vi "Oscilloscope.vi"() -> ()   [LabVIEW 2020]
uses:
  <vilib>/Utility/file.llb/Read Delimited Spreadsheet (DBL).vi
  <vilib>/express/express analysis/Spectral/Block/exnSpectralBlock spectral measurements RMS poly.vi
  <vilib>/express/express analysis/Spectral/Block/exnSpectralBlock spectral measurements RMS array WFM.vi
  <vilib>/express/express analysis/Spectral/XNode/ExpressSpectralMeasurementsBlockNode.xnode
panel:
  in  "Auto":bool
  in  "Amplitude/div":i32(knob)=10 scale=1.0..6.0
  in  "WAV Select":path
  in  "CSV Select":path
  in  "Save Image":bool
  in  "Channel":bool
  in  "High Cut Off":dbl(knob)=20000.0 min=1.0 scale=1.0..20000.0
  out "Moving Average Enable":bool
  in  "Moving Average Enable":bool
  in  "Moving Average\nWindow Size":u16(ring) items=["4", "8", "16"]
  in  "Reset":bool
  in  "Input Select":bool
  in  "stop":bool
  in  "Filter Order":i16(knob)=1 scale=1.0..5.0
  in  "Pause/Continue":bool
  in  "Tab Control":enum32{"Time", "FFT"}(tab)
  out "Waveform Chart":dbl(graph)
  out "Waveform Graph":cluster{"f0":dbl, "df":dbl, "magnitude":dbl[]}[](graph)
  in  "Period (ms)":dbl(knob)=10.0 scale=1.0..100.0
  out "Frequency (Hz)":dbl
  in  "Amplitude Control":dbl(knob)=1.0 min=1.0 scale=1.0..1000.0
  in  "Offset":i32(knob) scale=-10.0..10.0
  in  "Orig or not":bool=TRUE
  out "Original":bool
  in  "Filter or not":bool
  in  "Filter Select":u16(ring) items=["Lowpass", "Highpass", "Bandpass", "Bandstop", "Smoothing"]
  in  "Low Cut Off":dbl(knob)=1.0 min=1.0 scale=1.0..20000.0
  out "Filter Enable":bool
  in  "Phase Control":dbl(knob) scale=-360.0..360.0
  out "Pk-Pk":dbl
  out "RMS":dbl
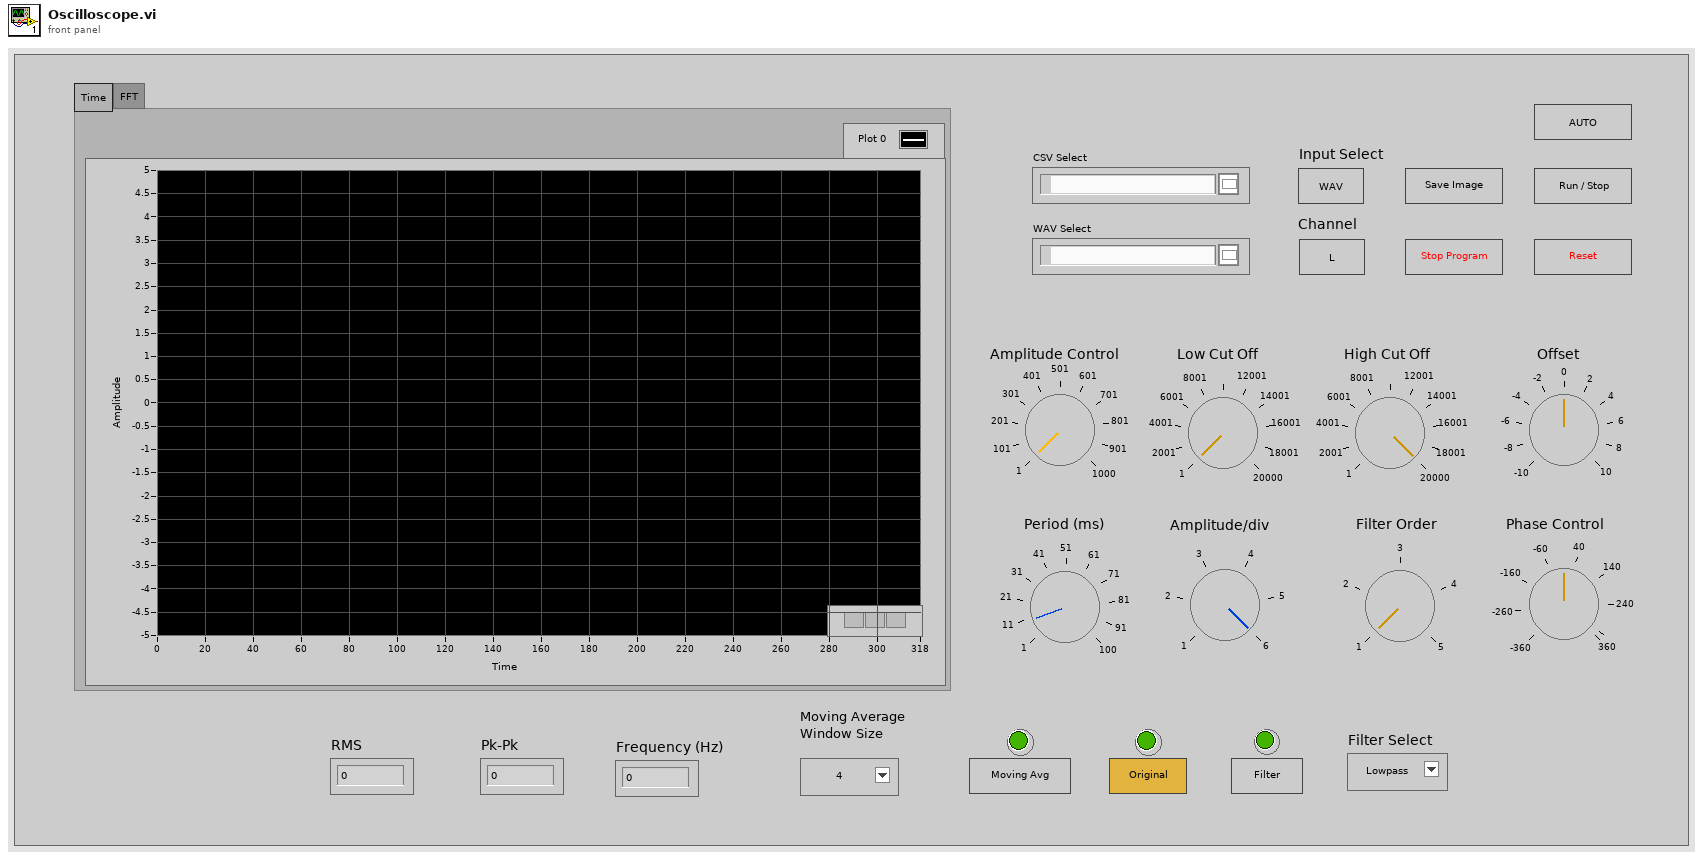
[diagram p1: front panel]
types:
  T1 = cluster{"averaging mode":u16, "weighting mode":u16, "number of averages":u32}
  T2 = cluster{"dB On (F)":bool, "unwrap phase (F)":bool, "convert to degree (F)":bool}
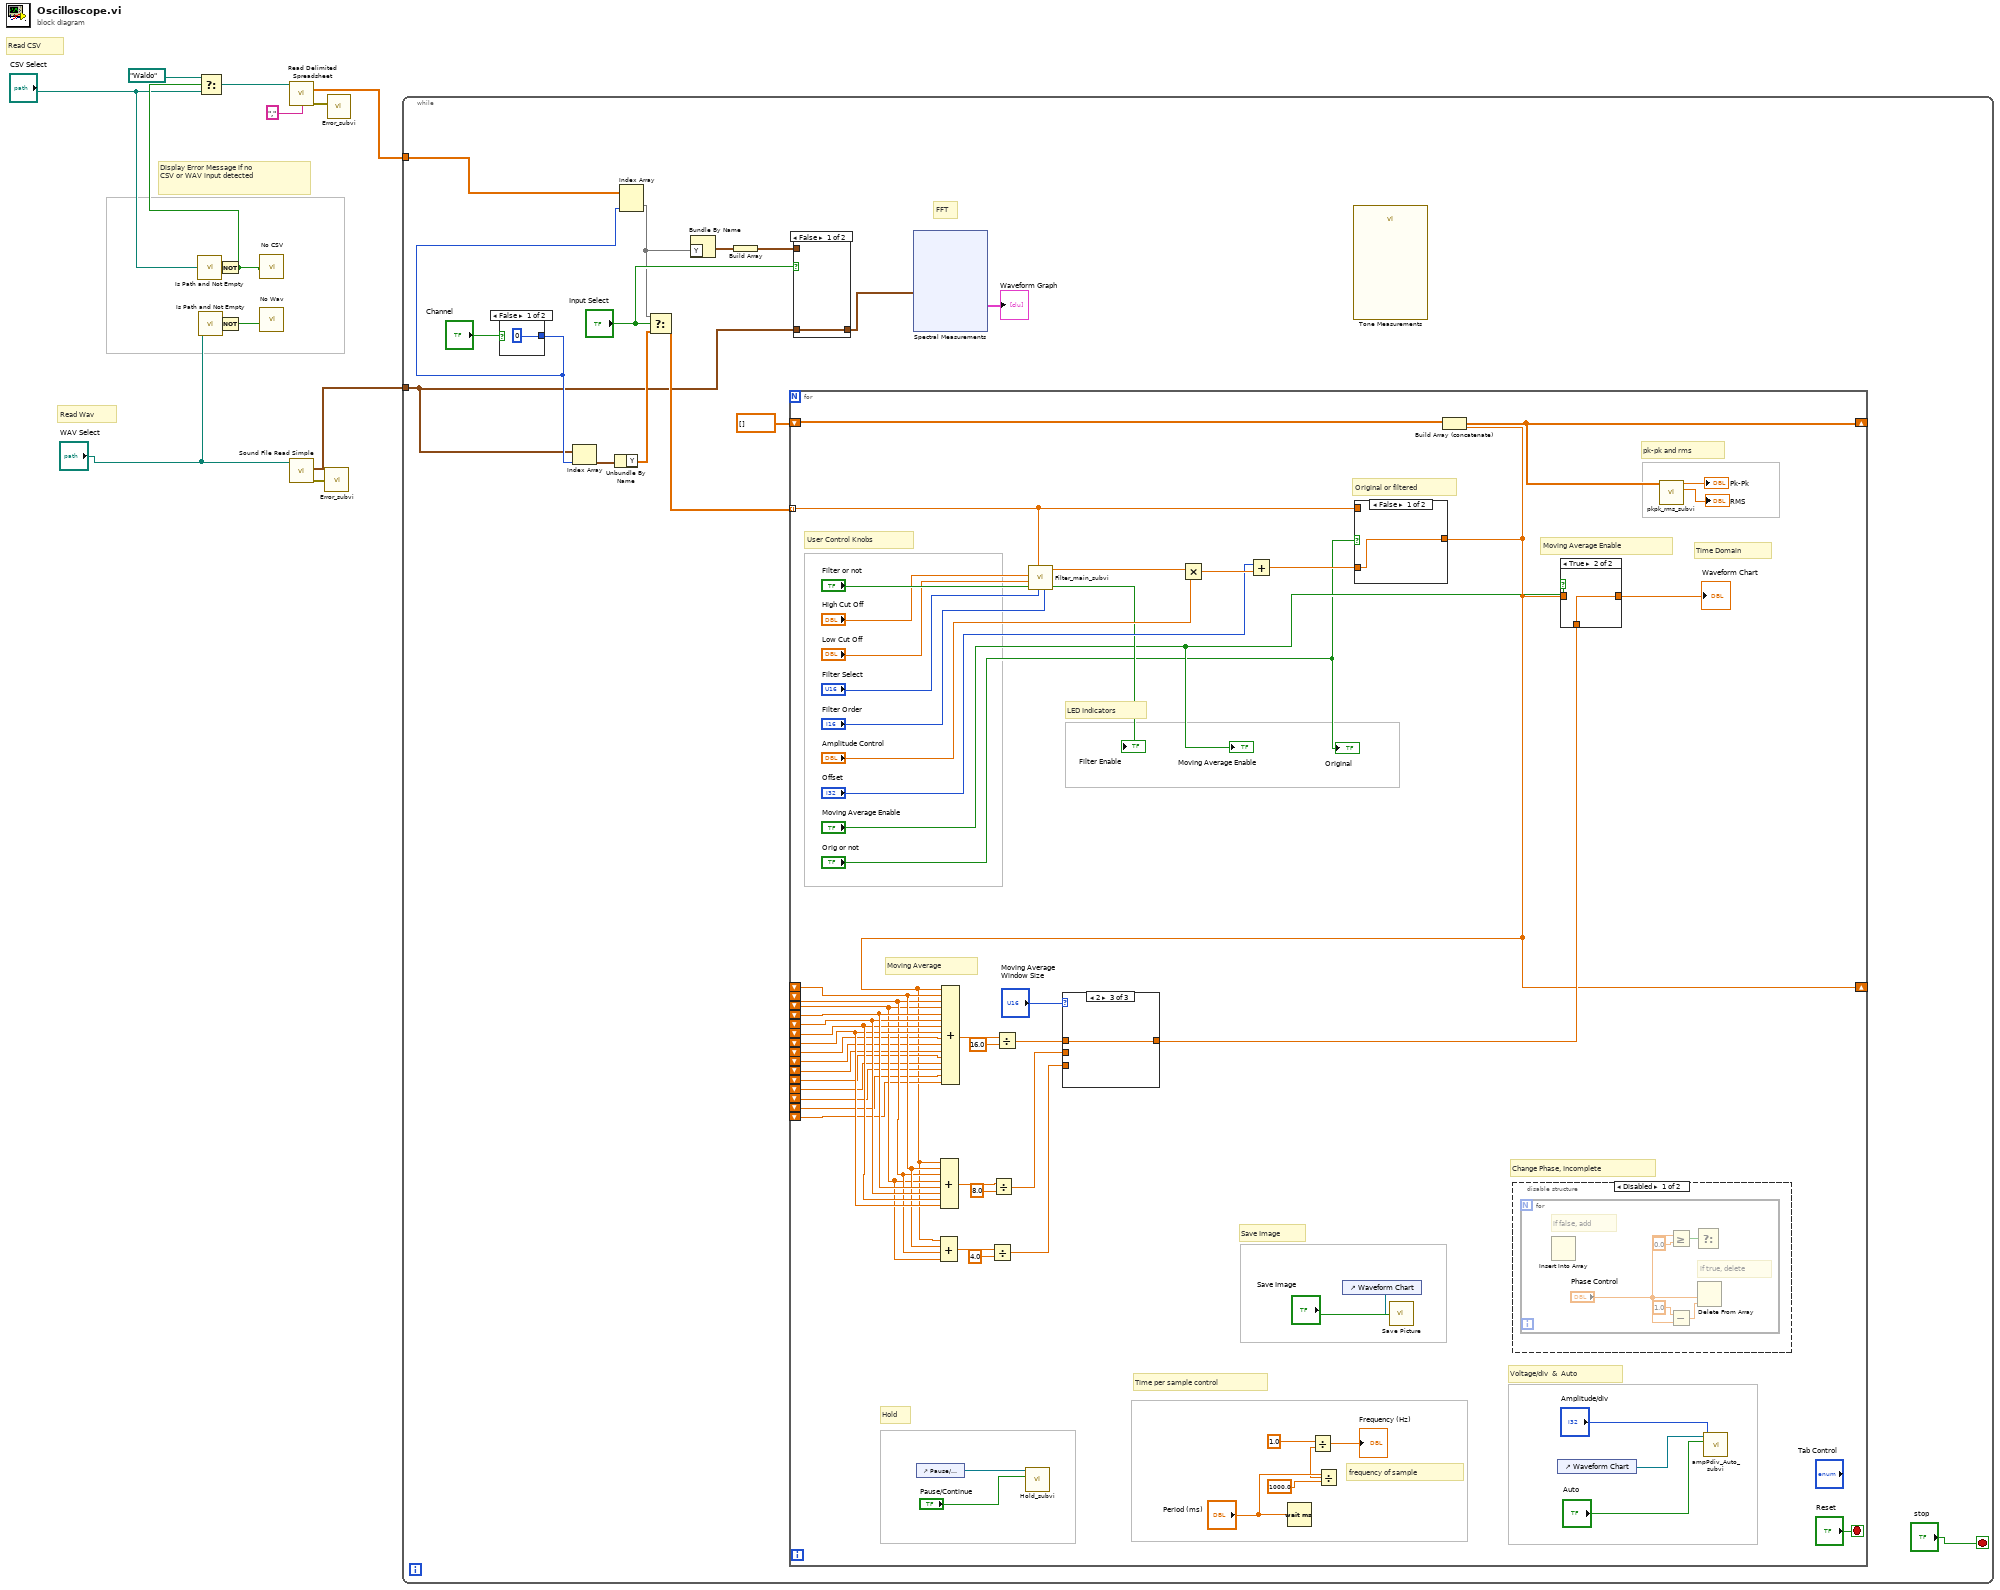
[diagram p0: block diagram]
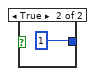
[diagram p3: hidden frame]
diagram:
  # "Display Error Message if no\nCSV or WAV input detected"
  # "Read CSV"
  # "Read Wav"
  n1 = call <vilib>:"Is Path and Not Empty.vi"("path"="CSV Select") -> ("Is Path and Not Empty?"=w8:bool)  [unwired: 4 in]
  n2 = call <vilib>:"Is Path and Not Empty.vi"("path"="WAV Select") -> ("Is Path and Not Empty?"=w9:bool)  [unwired: 4 in]
  n3 = Not(x=w8) -> (.not. x?=w4:bool)
  n4 = Select(t=path "Waldo", s=w4, f="CSV Select") -> (s? t:f=w3:path)
  n5 = Not(x=w9) -> (.not. x?=w7:bool)
  n6 = call "No CSV"("Enable"=w4) -> ()  [unwired: 9 in, 2 out]
  n7 = call "No Wav"("Enable"=w7) -> ()  [unwired: 9 in, 2 out]
  n8 = call-poly <vilib>:"Read Delimited Spreadsheet.vi"("file path (dialog if empty)"=w3, "delimiter (\\t)"="," ("delimiter (\\t)")) -> ("all rows"=w10:dbl[][], "error out"=w12:errorcluster)  [unwired: 8 in, 4 out]
  n9 = call <vilib>:"Sound File Read Simple.vi"("path"="WAV Select") -> ("error out"=w6:errorcluster, "data"=w13:waveform(dbl)[])  [unwired: 7 in, 2 out]
  n10 = call "Error_subvi.vi"("error in (no error)"=w6) -> ()  [unwired: 3 out]
  n11 = call "Error_subvi.vi"("error in (no error)"=w12) -> ()  [unwired: 3 out]
  n12 = while {
    tunnel: w13 -> [w20]
    tunnel: w10 -> [w19]
    stop <- "stop" stop-if-true
    # "FFT"
    n13 = case shown="False" "Channel" {
      tunnel: [0 ("index") 1 ("index")] -> w21
      frame False {
      }
      frame True {
      }
    }
    n14 = Index Array(array=w20, index=w21) -> (element=w27:waveform(dbl))
    n15 = Unbundle By Name(w27) -> ("Y"=w26:dbl[])
    n16 = Index Array(array=w19, index (col)=w21) -> (element=w23:dbl[])  [unwired: 1 in]
    n17 = Select(t=w23, s="Input Select", f=w26) -> (s? t:f=w25:dbl[])
    n18 = Bundle By Name("Y"=w23) -> (w15:waveform(dbl))  [unwired: 1 in]
    n19 = Build Array(w15) -> (w14:waveform(dbl)[])
    n20 = for {
      tunnel: w25 -> [w60] mode=indexing
      shift-right: [w93] -> _
      shift-left: dbl[] [] -> [w94]
      shift-right: [w65] -> _
      shift-left: _ -> [w86]
      shift-left: _ -> [w85]
      shift-left: _ -> [w84]
      shift-left: _ -> [w90]
      shift-left: _ -> [w89]
      shift-left: _ -> [w88]
      shift-left: _ -> [w87]
      shift-left: _ -> [w75]
      shift-left: _ -> [w74]
      shift-left: _ -> [w73]
      shift-left: _ -> [w72]
      shift-left: _ -> [w71]
      shift-left: _ -> [w70]
      shift-left: _ -> [w69]
      shift-left: _ -> [w68]
      stop <- "Reset" stop-if-true
      # "User Control Knobs"
      # "Original or filtered"
      # "Moving Average Enable"
      # "LED Indicators"
      # "pk-pk and rms"
      # "Save Image"
      # "Voltage/div  &  Auto"
      # "frequency of sample"
      # "Time per sample control"
      # "Moving Average"
      # "Hold"
      # "Time Domain"
      # "Change Phase, Incomplete"
      n21 = control-ref of="Pause/Continue"() -> (w48:refnum<vi>)
      n22 = call "Hold_subvi.vi"("Pause/Continue"="Pause/Continue", "Boolean in"=w48) -> ()  [unwired: 10 in]
      n23 = call "Filter_main_subvi.vi"("Filter Order"="Filter Order", "Filter Select"="Filter Select", "Numeric in"=w60, "Low Cut Off"="Low Cut Off", "High Cut Off"="High Cut Off", "Filter or not"="Filter or not") -> ("Numeric out"=w97:dbl)  [unwired: 5 in]
      n24 = Multiply(x=w97, y="Amplitude Control") -> (x*y=w99:dbl)
      n25 = Add(x="Offset", y=w99) -> (x+y=w96:dbl)
      n26 = Wait (ms)(milliseconds to wait="Period (ms)") -> ()  [unwired: 1 out]
      n27 = Divide(x="Period (ms)", y=1000.0 ("x")) -> (x/y=w56:dbl)
      n28 = Divide(x=1.0, y=w56) -> (x/y=→"Frequency (Hz)":dbl)
      n29 = control-ref of="Waveform Chart"() -> (w63:refnum<vi>)
      n30 = case shown="False" "Orig or not" {
        tunnel: w60 -> [_ w112]
        tunnel: [w111 w112] -> w65
        tunnel: w96 -> [w111 _]
        frame False {
        }
        frame True {
        }
      }
      n31 = Compound Arithmetic op=ADD(w65, w86, w85, w84) -> (w79:dbl)
      n32 = Compound Arithmetic op=ADD(w65, w86, w85, w84, w90, w89, w88, w87) -> (w81:dbl)
      n33 = Compound Arithmetic op=ADD(w65, w86, w85, w84, w90, w89, w88, w87, w75, w74, w73, w72, w71, w70, w69, w68) -> (w83:dbl)
      n34 = Divide(x=w79, y=4.0) -> (x/y=w53:dbl)
      n35 = Divide(x=w81, y=8.0) -> (x/y=w76:dbl)
      n36 = Divide(x=w83, y=16.0) -> (x/y=w77:dbl)
      n37 = case shown="2" "Moving Average\nWindow Size" {
        tunnel: w77 -> [_ _ w105]
        tunnel: w76 -> [_ w104 _]
        tunnel: w53 -> [w103 _ _]
        tunnel: [w103 w104 w105] -> w66
        frame 0, Default {
        }
        frame 1 {
        }
        frame 2 {
        }
      }
      n38 = call "Save Picture.vi"("Save Image"="Save Image", "WaveformChart in"=w63) -> ()
      n39 = Build Array (concatenate)(w94, w65) -> (w93:dbl[])
      n40 = disable-structure shown="Disabled" {
        frame Disabled {
          n41 = for {
            # "if false, add"
            # "if true, delete"
            n42 = Insert Into Array() -> ()  [unwired: 3 in, 1 out]
            n43 = Greater Or Equal?(x="Phase Control", y=0.0) -> (x >= y?=w109:bool)
            n44 = Subtract(x=1.0, y="Phase Control") -> (x-y=w106:dbl)
            n45 = Select(s=w109) -> ()  [unwired: 2 in, 1 out]
            n46 = Delete From Array(length="Phase Control", index=w106) -> ()  [unwired: 1 in, 2 out]
          }
        }
        frame Enabled {
        }
      }
      n47 = control-ref of="Waveform Chart"() -> (w47:refnum<vi>)
      n48 = case shown="True" "Moving Average Enable" {
        tunnel: w66 -> [_ w102]
        tunnel: [w101 w102] -> w59
        tunnel: w65 -> [w101 _]
        frame False {
        }
        frame True {
        }
      }
      "Waveform Chart" <- w59
      n49 = call "pkpk_rms_subvi.vi"("Array"=w93) -> ("RMS"=→"RMS":dbl, "Pk-Pk"=→"Pk-Pk":dbl)  [unwired: 9 in]
      n50 = call "ampPdiv_Auto_subvi.vi"("Amplitude/div"="Amplitude/div", "Auto"="Auto", "WaveformChart in"=w47) -> ()  [unwired: 9 in]
      "Original" <- "Orig or not"
      "Filter Enable" <- "Filter or not"
      "Moving Average Enable" <- "Moving Average Enable"
    }
    n51 = case shown="False" "Input Select" {
      tunnel: w20 -> [w29 _]
      tunnel: [w29 w30] -> w16
      tunnel: w14 -> [_ w30]
      frame False {
      }
      frame True {
      }
    }
    n52 = xnode "Spectral Measurements"("Signals"=w16) -> ("FFT - (RMS)"=→"Waveform Graph":cluster{"f0":dbl, "df":dbl, "magnitude":dbl[]}[])  [unwired: 1 in, 2 out]
    n53 = call "Tone Measurements"() -> ()  [unwired: 10 in, 2 out]
  }
